vi "traitement.vi"   [LabVIEW 2020]
uses:
  <vilib>/Utility/file.llb/Read Delimited Spreadsheet (DBL).vi
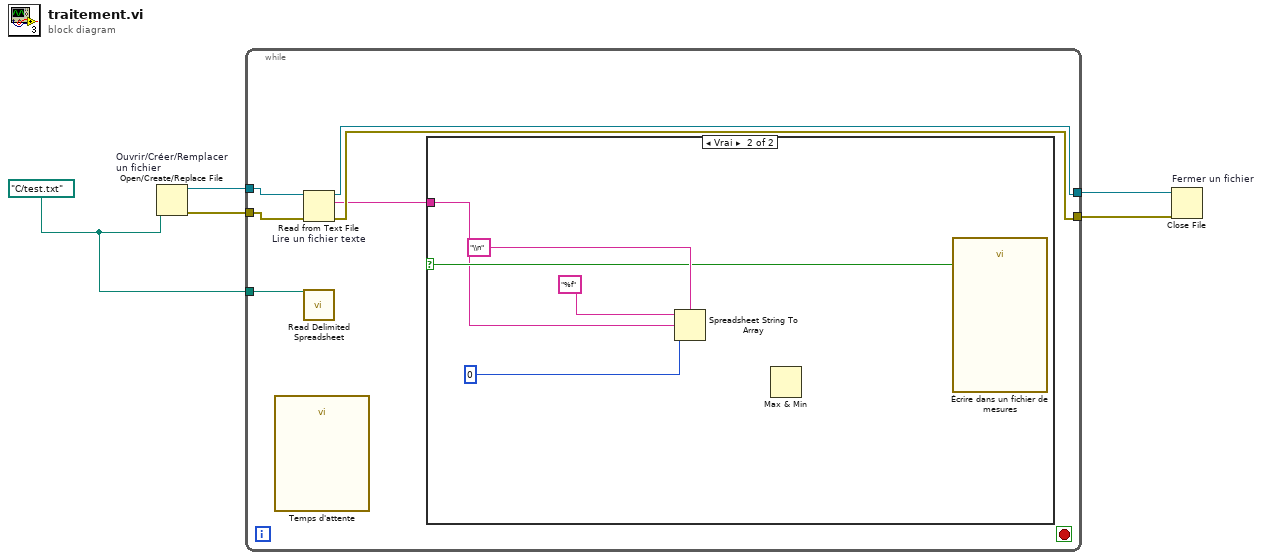
[diagram p0: block diagram]
diagram:
  w1 = path "C:/test.txt"
  n1 = Open/Create/Replace File "Ouvrir/Créer/Remplacer un fichier"(file path (use dialog)=w1) -> (refnum out=w5:refnum<file>, error out=w4:errorcluster)  [unwired: 5 in, 1 out]
  n2 = while {
    tunnel: w5 -> [w10]
    tunnel: w4 -> [w11]
    tunnel: [w7] -> w3
    tunnel: [w9] -> w2
    tunnel: w1 -> [w6]
    stop <- _ stop-if-true
    n3 = call "Temps d'attente"() -> ()  [unwired: 11 in, 1 out]
    n4 = Read from Text File "Lire un fichier texte"(file (use dialog)=w10, error in=w11) -> (refnum out=w7:refnum<file>, text=w8:string, error out=w9:errorcluster)  [unwired: 2 in, 1 out]
    n5 = call-poly <vilib>:"Read Delimited Spreadsheet.vi"("file path (dialog if empty)"=w6) -> ()  [unwired: 9 in, 6 out]
    n6 = case shown="Vrai" {
      selector: _ -> [_ w13]
      tunnel: w8 -> [_ w12]
      frame False {
      }
      frame True {
        n7 = Spreadsheet String To Array(delimiter (Tab)="\\n", format string="%f", spreadsheet string=w12, array type (2D Dbl)=0) -> ()  [unwired: 1 out]
        n8 = Max & Min() -> ()  [unwired: 2 in, 2 out]
        n9 = call "Écrire dans un fichier de mesures"("Enable"=w13) -> ()  [unwired: 16 in, 3 out]
      }
    }
  }
  n10 = Close File "Fermer un fichier"(refnum=w3, error in=w2) -> ()  [unwired: 2 out]
